vi "Main menu_3.vi"() -> ()   [LabVIEW 2022 SP3]
uses:
  <vilib>/event_ctls.llb/lveventtype.ctl
  <vilib>/Utility/file.llb/Write Delimited Spreadsheet (DBL).vi
panel:
  out "Waveform Chart 2":waveform(sgl)(graph)
  out "Waveform Chart":sgl[](graph)
  in  "# signal selec":string(combo)
  out "Close":bool
  in  "Close app":bool
  in  "?":T1(tab)
  in  "New plot":bool
  in  "Multicolumn Listbox":i32(listbox)
  in  "Close All plots":bool
  in  "CSV":bool
  in  "Start record":bool
  in  "Refresh \ntime (ms)":i32
  in  "Mode":enum32{"Item 0", "Item 1"}(radio)
  in  "Size bytes X #Traces":i32
  in  "Trace names":string(combo)
  in  "CTRL enable":bool
  in  "Save CTRL parameters":bool
  out "Total\ncontrols":i32
  in  "# Control":string(combo)
  in  "CS enable":bool
  out "Current CS status":i32
  in  "CS_IF_Params":T2 {"CS_Duty" min=0 max=1}
  out "Connected":bool
  out "Server Ping":string
  out "Saved":bool
  in  "Save conf":bool
  in  "Ping IP":bool
  in  "Port":i32
  in  "hostname":string
  in  "timeout ms":i32
  in  "Send message":bool
  in  "Process 2":i32
  in  "msj":string
  # "hostname: 127.0.0.1\nport: 8085"
  # "hostname\n131.246.75.169"
  # "Temporal for testing"
  # "Next activities:\n\n- Put preempt config in the from HW_\n- Continuos with refresh (share variable) _ temp"
  # "ctrl_if:0\nctrl: 2\nset parm: 2"
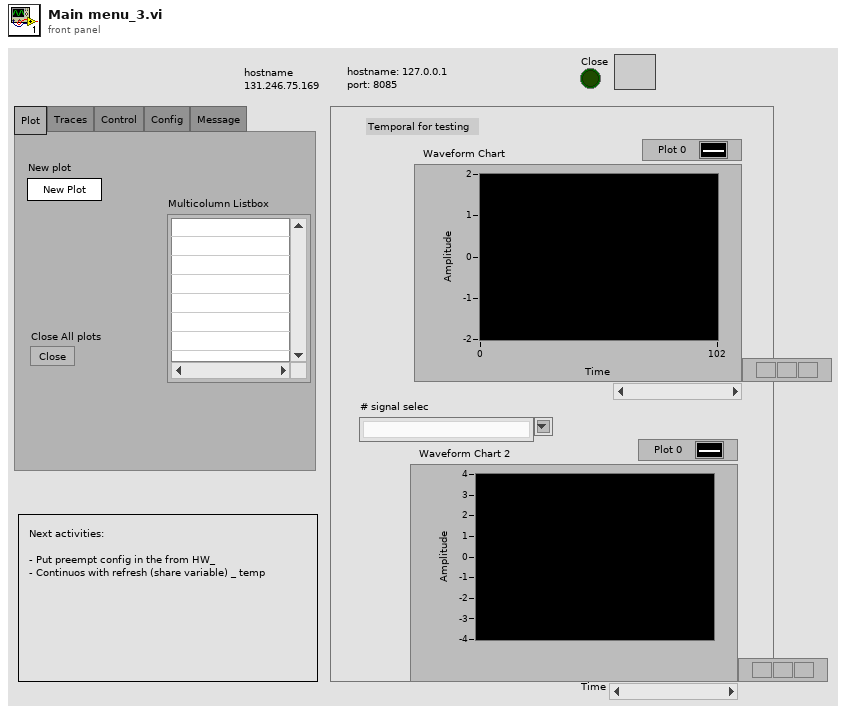
[diagram p1: front panel]
types:
  T1 = enum32{"Plot", "Traces", "Control", "Config", "Message"}
  T2 = cluster{"SET_PARAMETERS":i32, "CTLR":i32, "CS_Duty":sgl, "CTRL_IF_SET":i32}
  T3 = cluster{"Port":i32, "hostname":string, "status":bool, "timeout ms":i32, "TRACES_NAMES":string[], "Refresh time ms":i32, "Mode":enum32{"Item 0", "Item 1"}, "Start":bool, "DATA":sgl[][], "SIGNALS_NAMES":string[], "NB_SIGNALS":i32, "NB_TRACES":i32, "ID_TRACE":i32, "Mark":bool, "Counter":i32, "CTRLs_NAMES":string[], "NB_Ctrls":i32, "CS enable?":bool, "CS ID":i32}
  T4 = enum8{"Enabled", "Disabled", "Disabled and Grayed Out"}
  T5 = cluster{"TRACE_SIZE":i32, "CS_ID":i32, "TRACE ID":i32, "CMD":i32, "DATA PARAM":string}
  T6 = cluster{"TRACE_SIZE":i32, "CS_ID":i32, "TRACE ID":i32, "CMD":i32, "DATA(M)":i32}
  T7 = cluster{"timeout ms":i32, "remote port":u16, "Address":string}
  T8 = typedef "lveventtype.ctl" = enum32{"Null", "Timeout", "Annotation Menu Selection", "Annotation Menu Selection?", "App Instance Close", "App Instance Close?", "Autoscale Range Change", "Bookmark Info Change", "Cell Edit", "Cell Edit?", "Cursor Grab", "Cursor Grab?", "Cursor Menu Selection", "Cursor Menu Selection?", "Cursor Move", "Cursor Release", "Data Change", "Direction Change", "Display State Change", "Drag Ended", "Drag Enter", "Drag Leave", "Drag Over", "Drag Source Update", "Drag Starting", "Drag Starting?", "Drop", "Exec State Change", "Key Down", "Key Down?", "Key Repeat", "Key Repeat?", "Key Up", "Listbox Double Click", "Menu Activation?", "Menu Selection (App)", "Menu Selection? (App)", "Menu Selection (User)", "Mouse Down", "Mouse Down?", "Mouse Enter", "Mouse Leave", "Mouse Move", "Mouse Up", "Mouse Wheel", "NI Security User Change (App)", "Pane Size", "Panel Close", "Panel Close?", "Panel Resize", "Plot Attribute Change", "Scale Range Change", "Shortcut Menu Activation?", "Shortcut Menu Selection (App)", "Shortcut Menu Selection? (App)", "Shortcut Menu Selection (User)", "Tree Double Click", "Tree Drag", "Tree Drag?", "Tree Drop", "Tree Drop?", "Tree Item Close", "Tree Item Close?", "Tree Item Open", "Tree Item Open?", "User Event", "Value Change"}
  T9 = enum16{"open", "replace", "create", "open or create", "replace or create", "replace or create with confirmation"}
  T10 = enum16{"big-endian, network order", "native, host order", "little-endian"}
  T11 = cluster{"SIZE":i32, " TRACE DATA":sgl[], "TRACE_SIZE":i32, "NB_TRACES":i32, "NB_TRACED_SIGNALS":i32, "NAMES TRACED SIGNALS":string[], "NAMES TRACES":string[], "CS STATUS":i32, "NB_CSs":i32, "NAMES CSs":string[], "DATA (M)":sgl[], "CMD":i32}
  T12 = enum32{"invalid app kind", "Development System", "Run Time System", "Student Edition", "Embedded LabVIEW", "Evaluation", "Custom"}
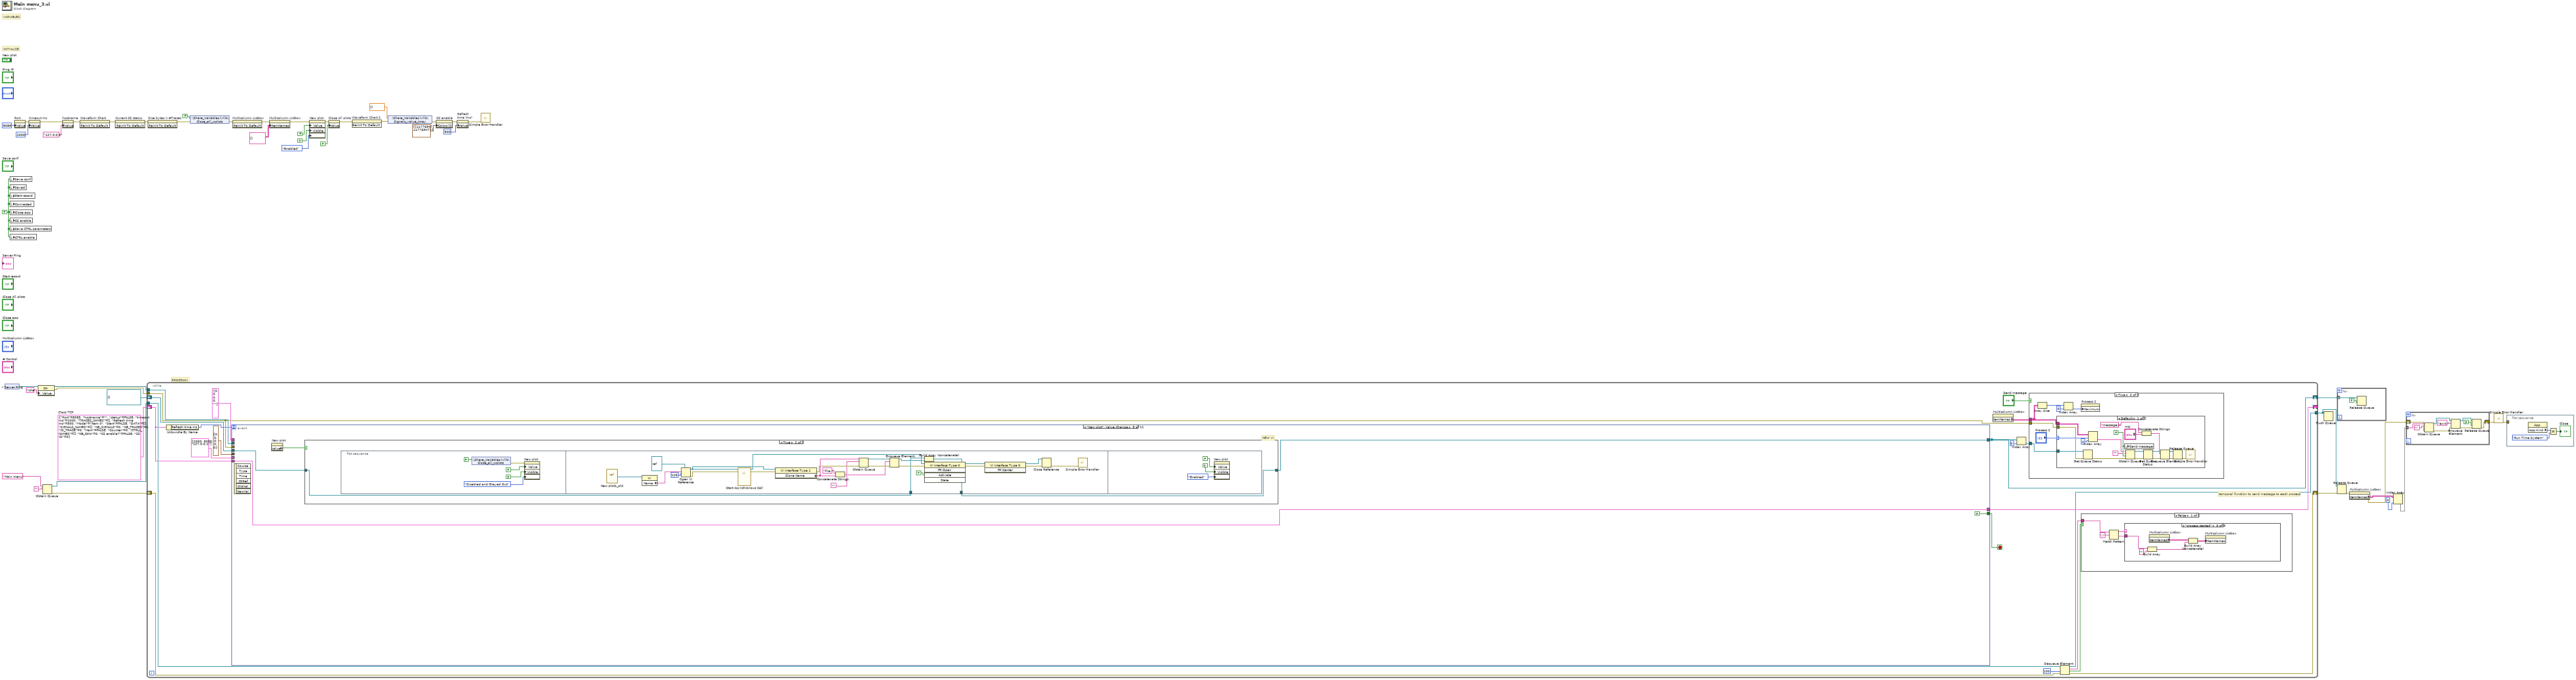
[diagram p0: block diagram]
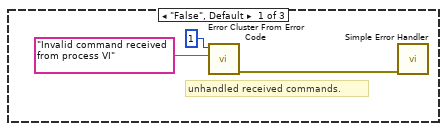
[diagram p4: hidden frame]
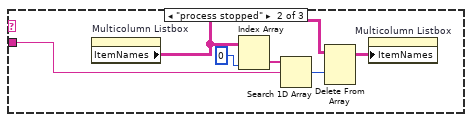
[diagram p5: hidden frame]
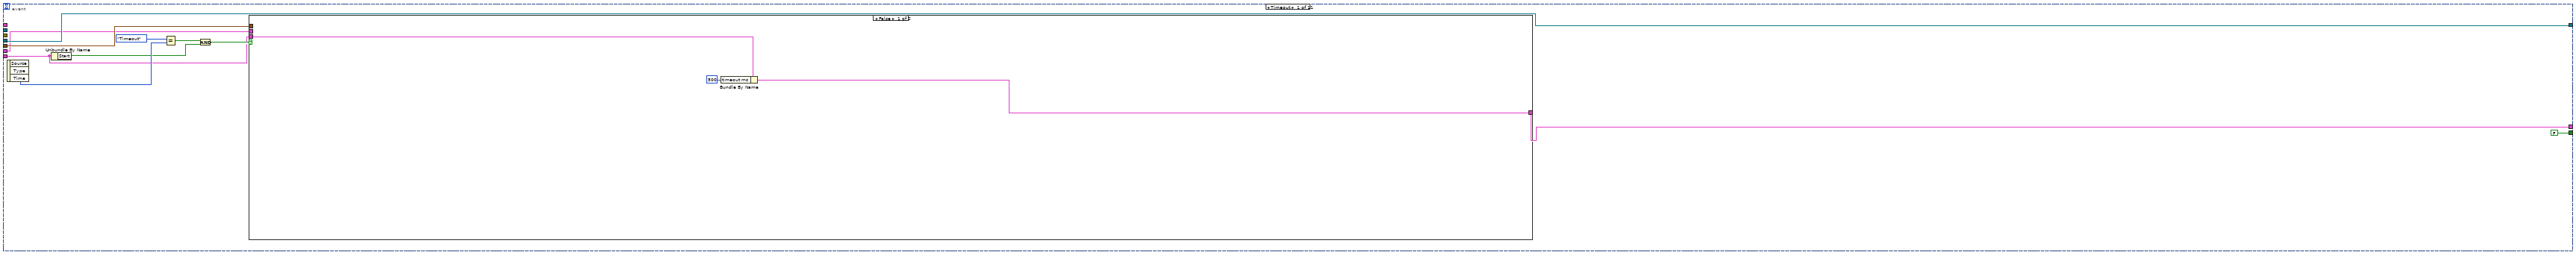
[diagram p7: hidden frame]
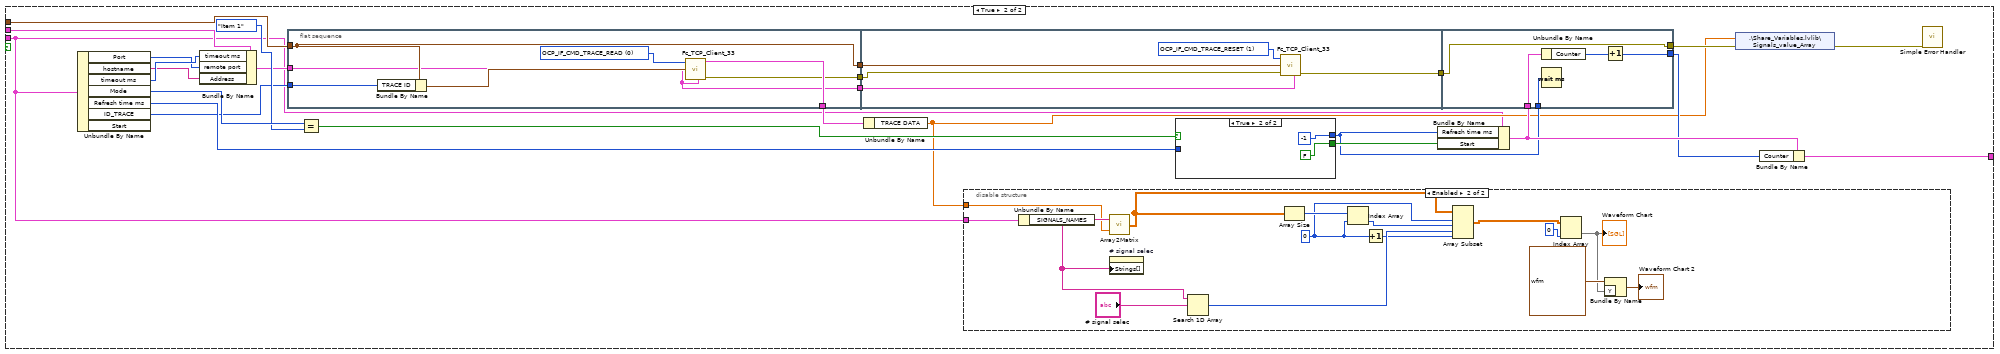
[diagram p8: hidden frame]
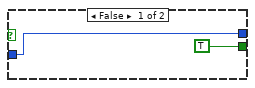
[diagram p10: hidden frame]
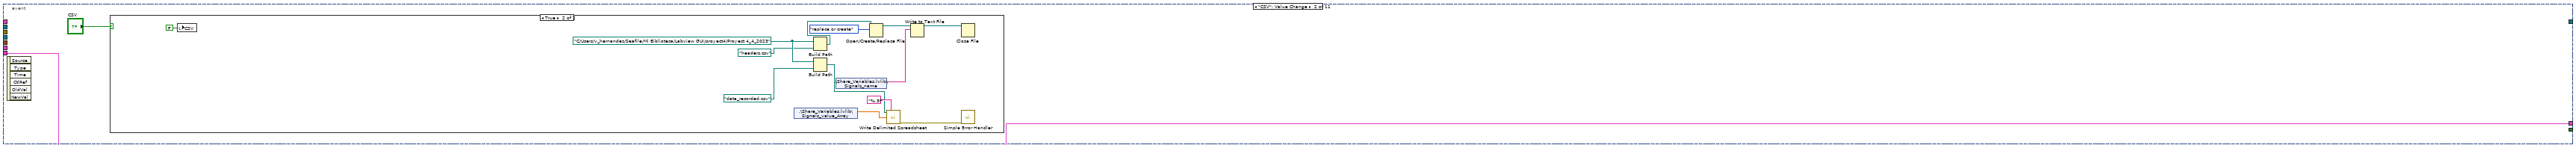
[diagram p11: hidden frame]
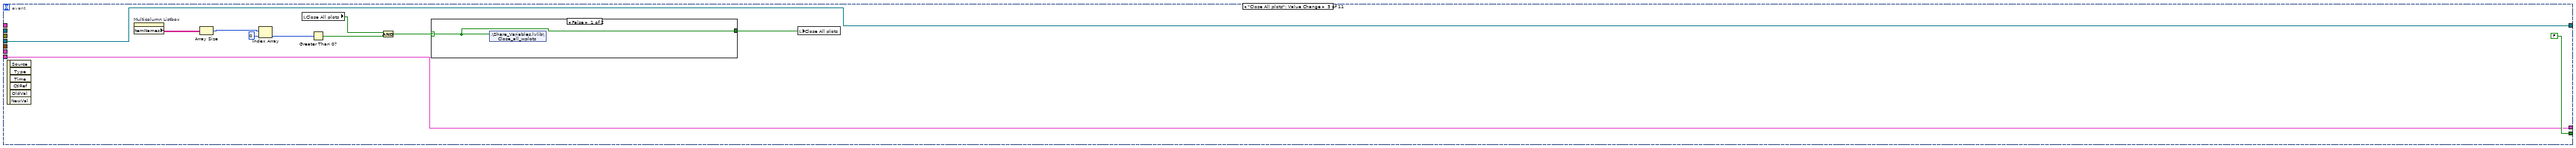
[diagram p13: hidden frame]
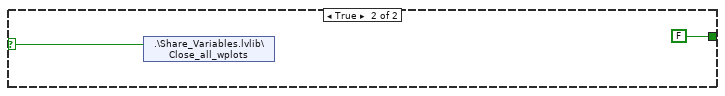
[diagram p14: hidden frame]
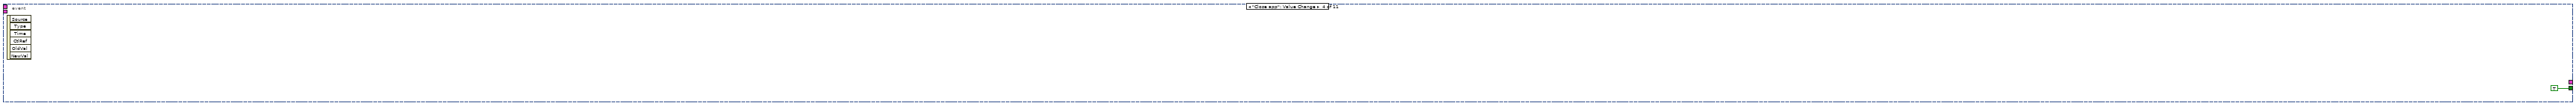
[diagram p15: hidden frame]
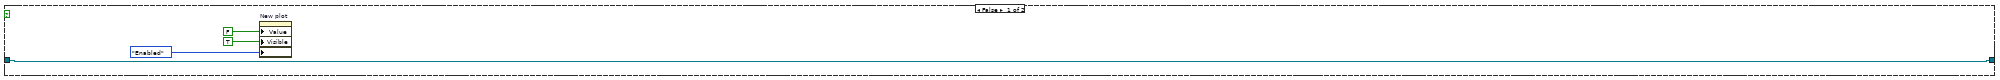
[diagram p16: hidden frame]
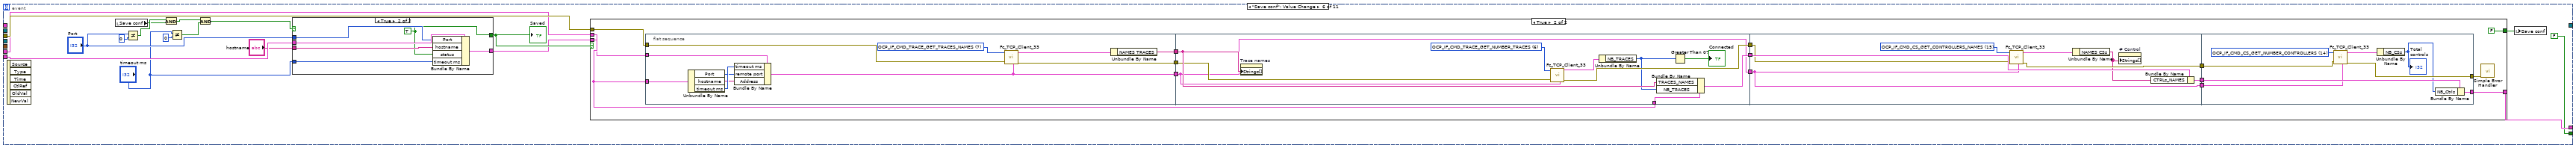
[diagram p17: hidden frame]
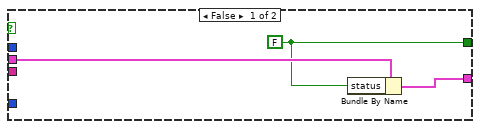
[diagram p19: hidden frame]
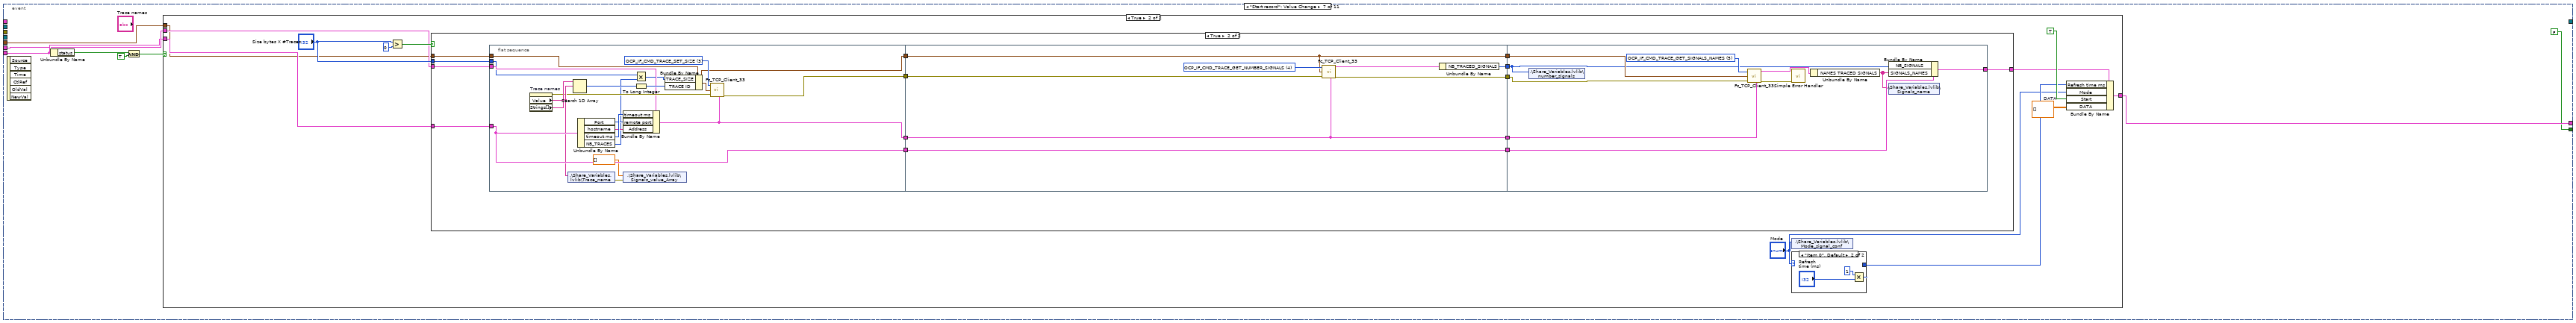
[diagram p20: hidden frame]
diagram:
  w26 = T3 {"Port"=8085, "hostname"="", "status"=FALSE, "timeout ms"=1000, "TRACES_NAMES"=[], "Refresh time ms"=500, "Mode"=enum."Item 0", "Start"=FALSE, "DATA"=[], "SIGNALS_NAMES"=[], "NB_SIGNALS"=0, "NB_TRACES"=0, "ID_TRACE"=0, "Mark"=FALSE, "Counter"=0, "CTRLs_NAMES"=[], "NB_Ctrls"=0, "CS enable?"=FALSE, "CS ID"=0}  # Class TCP
  w10 = FALSE ("Save conf")
  # "PROGRAM"
  # "INITIALIZE"
  # "VARIABLES"
  n1 = control-ref of="Server Ping"() -> (w23:refnum<vi>)
  n2 = local write "Save conf"(w10) -> ()
  n3 = local write "Saved"(w10) -> ()
  n4 = local write "Start record"(w10) -> ()
  n5 = local write "Connected"(w10) -> ()
  n6 = local write "Close app"(w10) -> ()
  n7 = local write "CS enable"(w10) -> ()
  n8 = local write "Save CTRL parameters"(w10) -> ()
  n9 = local write "CTRL enable"(w10) -> ()
  n10 = property on="Port" class="DigNum (strict)"("Value"=8085) -> (error out=w21:errorcluster)  [unwired: 2 in, 1 out]
  n11 = property on="timeout ms" class="DigNum (strict)"(error in=w21, "Value"=2000 ("timeout ms")) -> (error out=w17:errorcluster)  [unwired: 1 in, 1 out]
  n12 = property class="Str"(reference=w23, "Value"="Idle" ("Ping status")) -> (reference out=w25:refnum<vi>, error out=w24:errorcluster)  [unwired: 1 in]
  n13 = Obtain Queue(name (unnamed)="Main menu", element data type="") -> (queue out=w41:refnum<queue>, error out=w39:errorcluster)  [unwired: 3 in, 1 out]
  n14 = property on="hostname" class="Str"(error in=w17, "Value"="127.0.0.1" ("hostname")) -> (error out=w9:errorcluster)  [unwired: 1 in, 1 out]
  n15 = invoke on="Waveform Chart" class="WFChart (strict)" method="Reinit To Default"(error in=w9) -> (error out=w8:errorcluster)  [unwired: 2 in, 2 out]
  n16 = invoke on="Current CS status" class="DigNum (strict)" method="Reinit To Default"(error in=w8) -> (error out=w15:errorcluster)  [unwired: 2 in, 2 out]
  n17 = while {
    shift-right: [w53] -> w45
    shift-left: refnum<queue>[] [] -> [w69]
    tunnel: w41 -> [w68]
    tunnel: [w65] -> w31
    shift-right: [w58] -> w40
    shift-left: w39 -> [w64]
    shift-right: [w62] -> _
    shift-left: w26 -> [w60]
    tunnel: w25 -> [w61]
    tunnel: w24 -> [w55]
    stop <- w70 stop-if-true
    # "temporal function to send message to each process"
    n18 = Unbundle By Name(w60) -> ("Refresh time ms"=w59:i32)
    n19 = event shown="[4] \"New plot\": Value Change" {
      selector: _ -> [_ _ _ _ _ _ _ _ _ _ _]
      dyn-events: _ -> [_ _ _ _ _ _ _ _ _ _ _]
      timeout: w59 -> [_ _ _ _ _ _ _ _ _ _ _]
      tunnel: [FALSE ("f") _ FALSE ("f") TRUE ("f") FALSE ("f") FALSE ("f") FALSE ("f") FALSE ("f") _ _ _] -> w70
      tunnel: [w125 _ w215 _ w223 _ _ _ _ _ _] -> w53
      tunnel: w69 -> [w125 _ w215 _ w222 _ _ _ _ _ _]
      tunnel: [w118 w190 w205 _ w220 w271 w349 w423 w466 w531 w582] -> w62
      tunnel: w60 -> [w119 w190 w205 _ w220 w279 w350 w423 w465 w531 w582]
      tunnel: w61 -> [_ _ _ _ _ _ _ _ _ _ _]
      tunnel: w55 -> [_ _ _ _ _ w274 _ _ _ w532 w583]
      tunnel: T7 {"timeout ms"=2000, "remote port"=8085, "Address"="127.0.0.1"} ("Comunication Cluster") -> [w115 _ _ _ _ w264 w346 w427 w475 w528 w581]
      tunnel: T6 {"TRACE_SIZE"=0, "CS_ID"=0, "TRACE ID"=0, "CMD"=0, "DATA(M)"=0} ("Input Cluster") -> [w116 _ _ _ _ _ w345 w424 w474 _ _]
      tunnel: T5 {"TRACE_SIZE"=0, "CS_ID"=0, "TRACE ID"=0, "CMD"=0, "DATA PARAM"=""} ("Input Cluster") -> [_ _ _ _ _ _ _ _ _ w523 w576]
      event Timeout {
        n20 = event-data() -> ("Type"=w123:T8)  [unwired: 1 in, 2 out]
        n21 = Unbundle By Name(w119) -> ("Start"=w121:bool)
        n22 = Equal?(x=lveventtype."Timeout" ("Type"), y=w123) -> (x = y?=w122:bool)
        n23 = And(x=w122, y=w121) -> (x .and. y?=w120:bool)
        n24 = case shown="False" w120 {
          tunnel: w119 -> [w128 w129]
          tunnel: [w127 w143] -> w118
          tunnel: w116 -> [_ w132]
          tunnel: w115 -> [_ w131]
          frame False {
            n25 = Bundle By Name(cluster=w128, "timeout ms"=500) -> (w127:T3)
          }
          frame True {
            n26 = Unbundle By Name(w129) -> ("Port"=w137:i32, "hostname"=w136:string, "timeout ms"=w138:i32, "Mode"=w153:enum32{"Item 0", "Item 1"}, "Refresh time ms"=w150:i32, "ID_TRACE"=w147:i32)  [unwired: 1 out]
            n27 = Bundle By Name(cluster=w131, "timeout ms"=w138, "remote port"=w137, "Address"=w136) -> (w135:T7)
            n28 = flat-sequence {
              tunnel: w147 -> [w171]
              tunnel: [w175] -> w146
              tunnel: [w174] -> w145
              tunnel: w132 -> [w170]
              tunnel: [w170] -> w140
              tunnel: [w169] -> w139
              tunnel: w135 -> [w169]
              tunnel: w145 -> [w180]
              tunnel: w140 -> [w179]
              tunnel: w139 -> [w178]
              tunnel: [w176] -> w134
              tunnel: w144 -> [w185]
              tunnel: [w183] -> w142
              tunnel: w141 -> [w182]
              tunnel: w134 -> [w181]
              tunnel: [w181] -> w133
              frame #0 {
                w173 = 0 items=["OCP_IF_CMD_TRACE_READ", "OCP_IF_CMD_TRACE_RESET", "OCP_IF_CMD_TRACE_GET_SIZE", "OCP_IF_CMD_TRACE_SET_SIZE", "OCP_IF_CMD_TRACE_GET_NUMBER_SIGNALS", "OCP_IF_CMD_TRACE_GET_SIGNALS_NAMES", "OCP_IF_CMD_TRACE_GET_NUMBER_TRACES", "OCP_IF_CMD_TRACE_GET_TRACES_NAMES", "OCP_IF_CMD_TRACE_GET_ADDRESS", "OCP_IF_CMD_CS_STATUS", "OCP_IF_CMD_CS_ENABLE", "OCP_IF_CMD_CS_DISABLE", "OCP_IF_CMD_CS_CONTROLLER_IF", "OCP_IF_CMD_CS_HARDWARE_IF", "OCP_IF_CMD_CS_GET_NUMBER_CONTROLLERS", "OCP_IF_CMD_CS_GET_CONTROLLERS_NAMES", "OCP_IF_CMD_PLATFORM_ID", "OCP_IF_CMD_PLATFORM_IF", "OCP_IF_CMD_OPIL_UPDATE_MEASUREMENTS", "OCP_IF_CMD_OPIL_UPDATE_SIM_DATA", "OCP_IF_CMD_OPIL_RUN_CONTROL", "OCP_IF_CMD_OPIL_INITIALIZE_CONTROL", "OCP_IF_CMD_OPIL_GET_CONTROL", "OCP_IF_CMD_OPIL_GET_CONTROLLER_DATA", "OCP_IF_CMD_END"] ("CMD")
                n29 = Bundle By Name(cluster=w170, "TRACE ID"=w171) -> (w172:T6)
                n30 = call "Fc_TCP_Client_33.vi"("CMD"=w173, "Input Cluster"=w172, "Comunication Cluster"=w169) -> ("Output cluster"=w175:T11, "error out"=w174:errorcluster)  [unwired: 5 in, 1 out]
              }
              frame #1 {
                w177 = 1 items=["OCP_IF_CMD_TRACE_READ", "OCP_IF_CMD_TRACE_RESET", "OCP_IF_CMD_TRACE_GET_SIZE", "OCP_IF_CMD_TRACE_SET_SIZE", "OCP_IF_CMD_TRACE_GET_NUMBER_SIGNALS", "OCP_IF_CMD_TRACE_GET_SIGNALS_NAMES", "OCP_IF_CMD_TRACE_GET_NUMBER_TRACES", "OCP_IF_CMD_TRACE_GET_TRACES_NAMES", "OCP_IF_CMD_TRACE_GET_ADDRESS", "OCP_IF_CMD_CS_STATUS", "OCP_IF_CMD_CS_ENABLE", "OCP_IF_CMD_CS_DISABLE", "OCP_IF_CMD_CS_CONTROLLER_IF", "OCP_IF_CMD_CS_HARDWARE_IF", "OCP_IF_CMD_CS_GET_NUMBER_CONTROLLERS", "OCP_IF_CMD_CS_GET_CONTROLLERS_NAMES", "OCP_IF_CMD_PLATFORM_ID", "OCP_IF_CMD_PLATFORM_IF", "OCP_IF_CMD_OPIL_UPDATE_MEASUREMENTS", "OCP_IF_CMD_OPIL_UPDATE_SIM_DATA", "OCP_IF_CMD_OPIL_RUN_CONTROL", "OCP_IF_CMD_OPIL_INITIALIZE_CONTROL", "OCP_IF_CMD_OPIL_GET_CONTROL", "OCP_IF_CMD_OPIL_GET_CONTROLLER_DATA", "OCP_IF_CMD_END"] ("CMD")
                n31 = call "Fc_TCP_Client_33.vi"("CMD"=w177, "Input Cluster"=w179, "error in (no error)"=w180, "Comunication Cluster"=w178) -> ("error out"=w176:errorcluster)  [unwired: 4 in, 2 out]
              }
              frame #2 {
                n32 = Unbundle By Name(w185) -> ("Counter"=w184:i32)
                n33 = Wait (ms)(milliseconds to wait=w182) -> ()  [unwired: 1 out]
                n34 = Increment(x=w184) -> (x+1=w183:i32)
              }
            }
            n35 = Equal?(x=w153, y=enum32{"Item 0", "Item 1"}."Item 1" ("Mode")) -> (x = y?=w151:bool)
            n36 = Unbundle By Name(w146) -> ("TRACE DATA"=w130:sgl[])
            n37 = disable-structure shown="Enabled" {
              disable-tunnel: w130 -> [_ w164]
              disable-tunnel: w129 -> [_ w168]
              frame Disabled {
              }
              frame Enabled {
                w159 = 0 ("index")
                n38 = Unbundle By Name(w168) -> ("SIGNALS_NAMES"=w166:string[])
                n39 = call "Array2Matrix.vi"("Array"=w164, "Header"=w166) -> ("Array2D"=w163:sgl[][])
                n40 = property on="# signal selec" class="CmbBox"("Strings[]"=w166) -> ()  [unwired: 2 in, 2 out]
                n41 = Search 1D Array(1D array=w166, element="# signal selec") -> (index of element=w165:i32)  [unwired: 1 in]
                n42 = Array Size(array=w163) -> (size(s)=w162:i32[])
                n43 = Index Array(array=w162, index=w159) -> (element=w161:i32)
                n44 = Increment(x=w159) -> (x+1=w158:i32)
                n45 = Array Subset(array=w163, index (row)=w159, length (row)=w161, index (col)=w165, length (col)=w158) -> (w157:sgl[][])
                n46 = Index Array(array=w157, index (col)=0 ("disabled index (col)")) -> (element=w155:sgl[])  [unwired: 1 in]
                "Waveform Chart" <- w155
                n47 = Bundle By Name(cluster=waveform(sgl) {"t0"=timestamp(0 s since 1904-01-01), "dt"=1.0, "Y"=[]} ("waveform"), "Y"=w155) -> (→"Waveform Chart 2":waveform(sgl))
              }
            }
            n48 = case shown="True" w151 {
              tunnel: [TRUE FALSE] -> w149
              tunnel: [w186 i8 -1 ("t")] -> w141
              tunnel: w150 -> [w186 _]
              frame False {
              }
              frame True {
              }
            }
            n49 = Bundle By Name(cluster=w129, "Refresh time ms"=w141, "Start"=w149) -> (w144:T3)
            n50 = shared-variable ".\\Share_Variables.lvlib\\Signals_value_Array"(w130, error in=w133) -> (error out=w148:errorcluster)
            n51 = Bundle By Name(cluster=w144, "Counter"=w142) -> (w143:T3)
            n52 = call <vilib>:"Simple Error Handler.vi"("error in (no error)"=w148) -> ()  [unwired: 4 in, 5 out]
          }
        }
      }
      event "CSV": Value Change {
        n53 = event-data() -> ()  [unwired: 1 in, 6 out]
        n54 = case shown="True" "CSV" {
          frame False {
          }
          frame True {
            w199 = path "C:/Users/v_hernandez/Seafile/Mi Biblioteca/Labview GUI/proyect4/Proyect 4_4_2023" ("base path")
            n55 = local write "CSV"(FALSE ("CSV")) -> ()
            n56 = shared-variable ".\\Share_Variables.lvlib\\Signals_value_Array"() -> (w201:dbl[])  [unwired: 1 in, 1 out]
            n57 = Build Path(base path=w199, name or relative path=path "headers.csv") -> (appended path=w197:path)
            n58 = Build Path(base path=w199, name or relative path=path "data_recorded.csv") -> (appended path=w200:path)
            n59 = shared-variable ".\\Share_Variables.lvlib\\Signals_name"() -> (w194:string[])  [unwired: 1 in, 1 out]
            n60 = Open/Create/Replace File(file path (use dialog)=w197, operation (0:open)=T9."replace or create") -> (refnum out=w195:refnum<file>)  [unwired: 4 in, 2 out]
            n61 = call-poly <vilib>:"Write Delimited Spreadsheet.vi"("file path (dialog if empty)"=w200, "format (%.3f)"="%.3f", "1D data"=w201) -> ("error out"=w202:errorcluster)  [unwired: 11 in, 1 out]
            n62 = Write to Text File(file (use dialog)=w195, text=w194) -> (refnum out=w193:refnum<file>)  [unwired: 2 in, 2 out]
            n63 = Close File(refnum=w193) -> ()  [unwired: 1 in, 2 out]
            n64 = call <vilib>:"Simple Error Handler.vi"("error in (no error)"=w202) -> ()  [unwired: 4 in, 5 out]
          }
        }
      }
      event "Close All plots": Value Change {
        n65 = event-data() -> ()  [unwired: 1 in, 6 out]
        n66 = property on="Multicolumn Listbox" class="MCListbox (strict)"() -> ("ItemNames"=w209:string[][])  [unwired: 2 in, 2 out]
        n67 = Array Size(array=w209) -> (size(s)=w213:i32[])
        n68 = Index Array(array=w213, index=0) -> (element=w211:i32)
        n69 = local read "Close All plots"() -> (w208:bool)
        n70 = Greater Than 0?(x=w211) -> (x > 0?=w206:bool)
        n71 = And(x=w208, y=w206) -> (x .and. y?=w207:bool)
        n72 = case shown="False" w207 {
          selector: w207 -> [w216 w217]
          tunnel: [w216 FALSE] -> w210
          frame False {
            n73 = shared-variable ".\\Share_Variables.lvlib\\Close_all_wplots"(w216) -> ()  [unwired: 1 in, 1 out]
          }
          frame True {
            n74 = shared-variable ".\\Share_Variables.lvlib\\Close_all_wplots"(w217) -> ()  [unwired: 1 in, 1 out]
          }
        }
        n75 = local write "Close All plots"(w210) -> ()
      }
      event "Close app": Value Change {
        n76 = event-data() -> ()  [unwired: 1 in, 6 out]
      }
      event "New plot": Value Change {
        # "NEW VI"
        n77 = event-data() -> ()  [unwired: 1 in, 6 out]
        n78 = property on="New plot" class="Bool (strict)"() -> ("Value"=w224:bool)  [unwired: 2 in, 2 out]
        n79 = case shown="True" w224 {
          tunnel: [w225 w230] -> w223
          tunnel: w222 -> [w225 w229]
          frame False {
            n80 = property on="New plot" class="Bool (strict)"("Value"=FALSE ("New plot"), "Visible"=TRUE, "DisabledEnum"=T4."Enabled" ("Disabled")) -> ()  [unwired: 2 in, 2 out]
          }
          frame True {
            n81 = flat-sequence {
              tunnel: [w241] -> w230
              tunnel: w229 -> [w240]
              frame #0 {
                n82 = shared-variable ".\\Share_Variables.lvlib\\Close_all_wplots"(FALSE ("Close_all_wplots")) -> (error out=w231:errorcluster)  [unwired: 1 in]
                n83 = property on="New plot" class="Bool (strict)"(error in=w231, "Value"=FALSE ("New plot"), "Visible"=FALSE, "DisabledEnum"=T4."Disabled and Grayed Out" ("Disabled")) -> ()  [unwired: 1 in, 2 out]
              }
              frame #1 {
                n84 = vi-ref "New plot1_old.vi"() -> (w254:refnum<vi>)
                n85 = property class="VI"(reference=w254) -> ("Name"=w260:string)  [unwired: 1 in, 2 out]
                n86 = Open VI Reference(type specifier VI Refnum (for type only)=refnum<vi> refnum, vi path=w260, options=128) -> (vi reference=w251:refnum<vi>, error out=w256:errorcluster)  [unwired: 3 in]
                n87 = call-by-ref "Start Asynchronous Call"(reference=w251, error in=w256) -> (reference out=w255:refnum<vi>, error out=w245:errorcluster)  [unwired: 1 in, 1 out]
                n88 = property class="VI Interface Type 1"(reference=w251, error in=w245) -> (error out=w246:errorcluster, "Clone Name"=w248:string)  [unwired: 1 out]
                n89 = Concatenate Strings("file::" ("string"), w248) -> (w239:string)
                n90 = Obtain Queue(name (unnamed)=w248, element data type="", error in (no error)=w246) -> (queue out=w247:refnum<queue>, error out=w244:errorcluster)  [unwired: 2 in, 1 out]
                n91 = Enqueue Element(queue=w247, element=w239, error in (no error)=w244) -> (queue out=w242:refnum<queue>, error out=w243:errorcluster)  [unwired: 1 in, 1 out]
                n92 = Build Array (concatenate)(w240, w242) -> (w241:refnum<queue>[])
                n93 = invoke class="VI Interface Type 0" method="FP.Open"(reference=w255, error in=w243, "Activate"=TRUE ("Activate?")) -> (reference out=w253:refnum<vi>, error out=w238:errorcluster)  [unwired: 2 in, 3 out]
                n94 = invoke class="VI Interface Type 0" method="FP.Center"(reference=w253, error in=w238) -> (reference out=w252:refnum<vi>, error out=w237:errorcluster)  [unwired: 1 in, 1 out]
                n95 = Close Reference(reference=w252, error in (no error)=w237) -> (error out=w236:errorcluster)
                n96 = call <vilib>:"Simple Error Handler.vi"("error in (no error)"=w236) -> ()  [unwired: 4 in, 5 out]
              }
              frame #2 {
                n97 = property on="New plot" class="Bool (strict)"("Value"=FALSE ("Value (Signaling)"), "Visible"=TRUE, "DisabledEnum"=T4."Enabled" ("Disabled")) -> ()  [unwired: 2 in, 2 out]
              }
            }
          }
        }
      }
      event "Save conf": Value Change {
        n98 = event-data() -> ()  [unwired: 1 in, 6 out]
        n99 = local read "Save conf"() -> (w276:bool)
        n100 = Not Equal?(x="Port", y=0) -> (x != y?=w280:bool)
        n101 = And(x=w280, y=w276) -> (x .and. y?=w266:bool)
        n102 = Not Equal?(x="timeout ms", y=0) -> (x != y?=w268:bool)
        n103 = And(x=w266, y=w268) -> (x .and. y?=w267:bool)
        n104 = case shown="True" w267 {
          tunnel: [w336 w341] -> w275
          tunnel: "Port" -> [_ w343]
          tunnel: "hostname" -> [_ w342]
          tunnel: [w338 w339] -> w272
          tunnel: w279 -> [w337 w344]
          tunnel: "timeout ms" -> [_ w340]
          frame False {
            w336 = FALSE
            n105 = Bundle By Name(cluster=w337, "status"=w336) -> (w338:T3)
          }
          frame True {
            w341 = TRUE
            n106 = Bundle By Name(cluster=w344, "Port"=w343, "hostname"=w342, "status"=w341, "timeout ms"=w340) -> (w339:T3)
          }
        }
        "Saved" <- w275
        n107 = case shown="True" w275 {
          selector: w275 -> [w282 _]
          tunnel: w274 -> [_ w286]
          tunnel: [w282 FALSE] -> w273
          tunnel: w272 -> [w283 w297]
          tunnel: [w283 w296] -> w271
          tunnel: w264 -> [_ w284]
          frame False {
          }
          frame True {
            n108 = flat-sequence {
              tunnel: w297 -> [w309]
              tunnel: [w303] -> w295
              tunnel: [w302] -> w294
              tunnel: [w301] -> w293
              tunnel: w286 -> [w300]
              tunnel: w284 -> [w299]
              tunnel: w297 -> [w319]
              tunnel: w295 -> [w317]
              tunnel: w294 -> [w316]
              tunnel: w293 -> [w312]
              tunnel: [w318] -> w292
              tunnel: [w313] -> w290
              tunnel: [w312] -> w289
              tunnel: w292 -> [w327]
              tunnel: [w321] -> w291
              tunnel: w290 -> [w326]
              tunnel: w289 -> [w323]
              tunnel: [w324] -> w288
              tunnel: [w323] -> w287
              tunnel: [w331] -> w296
              tunnel: w291 -> [w335]
              tunnel: w288 -> [w334]
              tunnel: w287 -> [w333]
              tunnel: [w329] -> w285
              frame #0 {
                w308 = 7 items=["OCP_IF_CMD_TRACE_READ", "OCP_IF_CMD_TRACE_RESET", "OCP_IF_CMD_TRACE_GET_SIZE", "OCP_IF_CMD_TRACE_SET_SIZE", "OCP_IF_CMD_TRACE_GET_NUMBER_SIGNALS", "OCP_IF_CMD_TRACE_GET_SIGNALS_NAMES", "OCP_IF_CMD_TRACE_GET_NUMBER_TRACES", "OCP_IF_CMD_TRACE_GET_TRACES_NAMES", "OCP_IF_CMD_TRACE_GET_ADDRESS", "OCP_IF_CMD_CS_STATUS", "OCP_IF_CMD_CS_ENABLE", "OCP_IF_CMD_CS_DISABLE", "OCP_IF_CMD_CS_CONTROLLER_IF", "OCP_IF_CMD_CS_HARDWARE_IF", "OCP_IF_CMD_CS_GET_NUMBER_CONTROLLERS", "OCP_IF_CMD_CS_GET_CONTROLLERS_NAMES", "OCP_IF_CMD_PLATFORM_ID", "OCP_IF_CMD_PLATFORM_IF", "OCP_IF_CMD_OPIL_UPDATE_MEASUREMENTS", "OCP_IF_CMD_OPIL_UPDATE_SIM_DATA", "OCP_IF_CMD_OPIL_RUN_CONTROL", "OCP_IF_CMD_OPIL_INITIALIZE_CONTROL", "OCP_IF_CMD_OPIL_GET_CONTROL", "OCP_IF_CMD_OPIL_GET_CONTROLLER_DATA", "OCP_IF_CMD_END"] ("CMD")
                n109 = Unbundle By Name(w309) -> ("Port"=w305:i32, "hostname"=w304:string, "timeout ms"=w306:i32)
                n110 = Bundle By Name(cluster=w299, "timeout ms"=w306, "remote port"=w305, "Address"=w304) -> (w301:T7)
                n111 = call "Fc_TCP_Client_33.vi"("CMD"=w308, "error in (no error)"=w300, "Comunication Cluster"=w301) -> ("Output cluster"=w307:T11, "error out"=w302:errorcluster)  [unwired: 5 in, 1 out]
                n112 = Unbundle By Name(w307) -> ("NAMES TRACES"=w303:string[])
              }
              frame #1 {
                w315 = 6 items=["OCP_IF_CMD_TRACE_READ", "OCP_IF_CMD_TRACE_RESET", "OCP_IF_CMD_TRACE_GET_SIZE", "OCP_IF_CMD_TRACE_SET_SIZE", "OCP_IF_CMD_TRACE_GET_NUMBER_SIGNALS", "OCP_IF_CMD_TRACE_GET_SIGNALS_NAMES", "OCP_IF_CMD_TRACE_GET_NUMBER_TRACES", "OCP_IF_CMD_TRACE_GET_TRACES_NAMES", "OCP_IF_CMD_TRACE_GET_ADDRESS", "OCP_IF_CMD_CS_STATUS", "OCP_IF_CMD_CS_ENABLE", "OCP_IF_CMD_CS_DISABLE", "OCP_IF_CMD_CS_CONTROLLER_IF", "OCP_IF_CMD_CS_HARDWARE_IF", "OCP_IF_CMD_CS_GET_NUMBER_CONTROLLERS", "OCP_IF_CMD_CS_GET_CONTROLLERS_NAMES", "OCP_IF_CMD_PLATFORM_ID", "OCP_IF_CMD_PLATFORM_IF", "OCP_IF_CMD_OPIL_UPDATE_MEASUREMENTS", "OCP_IF_CMD_OPIL_UPDATE_SIM_DATA", "OCP_IF_CMD_OPIL_RUN_CONTROL", "OCP_IF_CMD_OPIL_INITIALIZE_CONTROL", "OCP_IF_CMD_OPIL_GET_CONTROL", "OCP_IF_CMD_OPIL_GET_CONTROLLER_DATA", "OCP_IF_CMD_END"] ("CMD")
                n113 = property on="Trace names" class="CmbBox"("Strings[]"=w317) -> ()  [unwired: 2 in, 2 out]
                n114 = call "Fc_TCP_Client_33.vi"("CMD"=w315, "error in (no error)"=w316, "Comunication Cluster"=w312) -> ("Output cluster"=w314:T11, "error out"=w313:errorcluster)  [unwired: 5 in, 1 out]
                n115 = Unbundle By Name(w314) -> ("NB_TRACES"=w311:i32)
                n116 = Bundle By Name(cluster=w319, "TRACES_NAMES"=w317, "NB_TRACES"=w311) -> (w318:T3)
                n117 = Greater Than 0?(x=w311) -> (x > 0?=→"Connected":bool)
              }
              frame #2 {
                w325 = 15 items=["OCP_IF_CMD_TRACE_READ", "OCP_IF_CMD_TRACE_RESET", "OCP_IF_CMD_TRACE_GET_SIZE", "OCP_IF_CMD_TRACE_SET_SIZE", "OCP_IF_CMD_TRACE_GET_NUMBER_SIGNALS", "OCP_IF_CMD_TRACE_GET_SIGNALS_NAMES", "OCP_IF_CMD_TRACE_GET_NUMBER_TRACES", "OCP_IF_CMD_TRACE_GET_TRACES_NAMES", "OCP_IF_CMD_TRACE_GET_ADDRESS", "OCP_IF_CMD_CS_STATUS", "OCP_IF_CMD_CS_ENABLE", "OCP_IF_CMD_CS_DISABLE", "OCP_IF_CMD_CS_CONTROLLER_IF", "OCP_IF_CMD_CS_HARDWARE_IF", "OCP_IF_CMD_CS_GET_NUMBER_CONTROLLERS", "OCP_IF_CMD_CS_GET_CONTROLLERS_NAMES", "OCP_IF_CMD_PLATFORM_ID", "OCP_IF_CMD_PLATFORM_IF", "OCP_IF_CMD_OPIL_UPDATE_MEASUREMENTS", "OCP_IF_CMD_OPIL_UPDATE_SIM_DATA", "OCP_IF_CMD_OPIL_RUN_CONTROL", "OCP_IF_CMD_OPIL_INITIALIZE_CONTROL", "OCP_IF_CMD_OPIL_GET_CONTROL", "OCP_IF_CMD_OPIL_GET_CONTROLLER_DATA", "OCP_IF_CMD_END"] ("CMD")
                n118 = call "Fc_TCP_Client_33.vi"("CMD"=w325, "error in (no error)"=w326, "Comunication Cluster"=w323) -> ("Output cluster"=w322:T11, "error out"=w324:errorcluster)  [unwired: 5 in, 1 out]
                n119 = Unbundle By Name(w322) -> ("NAMES CSs"=w320:string[])
                n120 = property on="# Control" class="CmbBox"("Strings[]"=w320) -> ()  [unwired: 2 in, 2 out]
                n121 = Bundle By Name(cluster=w327, "CTRLs_NAMES"=w320) -> (w321:T3)
              }
              frame #3 {
                w332 = 14 items=["OCP_IF_CMD_TRACE_READ", "OCP_IF_CMD_TRACE_RESET", "OCP_IF_CMD_TRACE_GET_SIZE", "OCP_IF_CMD_TRACE_SET_SIZE", "OCP_IF_CMD_TRACE_GET_NUMBER_SIGNALS", "OCP_IF_CMD_TRACE_GET_SIGNALS_NAMES", "OCP_IF_CMD_TRACE_GET_NUMBER_TRACES", "OCP_IF_CMD_TRACE_GET_TRACES_NAMES", "OCP_IF_CMD_TRACE_GET_ADDRESS", "OCP_IF_CMD_CS_STATUS", "OCP_IF_CMD_CS_ENABLE", "OCP_IF_CMD_CS_DISABLE", "OCP_IF_CMD_CS_CONTROLLER_IF", "OCP_IF_CMD_CS_HARDWARE_IF", "OCP_IF_CMD_CS_GET_NUMBER_CONTROLLERS", "OCP_IF_CMD_CS_GET_CONTROLLERS_NAMES", "OCP_IF_CMD_PLATFORM_ID", "OCP_IF_CMD_PLATFORM_IF", "OCP_IF_CMD_OPIL_UPDATE_MEASUREMENTS", "OCP_IF_CMD_OPIL_UPDATE_SIM_DATA", "OCP_IF_CMD_OPIL_RUN_CONTROL", "OCP_IF_CMD_OPIL_INITIALIZE_CONTROL", "OCP_IF_CMD_OPIL_GET_CONTROL", "OCP_IF_CMD_OPIL_GET_CONTROLLER_DATA", "OCP_IF_CMD_END"] ("CMD")
                n122 = call "Fc_TCP_Client_33.vi"("CMD"=w332, "error in (no error)"=w334, "Comunication Cluster"=w333) -> ("Output cluster"=w330:T11, "error out"=w329:errorcluster)  [unwired: 5 in, 1 out]
                n123 = Unbundle By Name(w330) -> ("NB_CSs"=w328:i32)
                "Total\ncontrols" <- w328
                n124 = Bundle By Name(cluster=w335, "NB_Ctrls"=w328) -> (w331:T3)
              }
            }
            n125 = call <vilib>:"Simple Error Handler.vi"("error in (no error)"=w285) -> ()  [unwired: 4 in, 5 out]
          }
        }
        n126 = local write "Save conf"(w273) -> ()
      }
      event "Start record": Value Change {
        n127 = event-data() -> ()  [unwired: 1 in, 6 out]
        n128 = Unbundle By Name(w350) -> ("status"=w352:bool)
        n129 = And(x=w352, y=TRUE) -> (x .and. y?=w351:bool)
        n130 = case shown="True" w351 {
          tunnel: w350 -> [w353 w359]
          tunnel: [w353 w365] -> w349
          tunnel: w346 -> [_ w356]
          tunnel: w345 -> [_ w355]
          frame False {
          }
          frame True {
            w354 = sgl[][] []  # DATA
            n131 = Greater?(x="Size bytes X #Traces", y=0) -> (0:w361:bool)
            n132 = case shown="True" w361 {
              tunnel: "Size bytes X #Traces" -> [_ w380]
              tunnel: w359 -> [w366 w379]
              tunnel: [w366 w375] -> w358
              tunnel: w356 -> [_ w368]
              tunnel: w355 -> [_ w367]
              frame False {
              }
              frame True {
                n133 = flat-sequence {
                  tunnel: w380 -> [w384]
                  tunnel: w379 -> [w400]
                  tunnel: [w396] -> w378
                  tunnel: [w400] -> w377
                  tunnel: [w389] -> w374
                  tunnel: [w388] -> w373
                  tunnel: w368 -> [w387]
                  tunnel: w367 -> [w386]
                  tunnel: w378 -> [w407]
                  tunnel: w377 -> [w408]
                  tunnel: [w408] -> w376
                  tunnel: w374 -> [w401]
                  tunnel: w373 -> [w402]
                  tunnel: [w404] -> w372
                  tunnel: [w403] -> w371
                  tunnel: [w402] -> w370
                  tunnel: [w401] -> w369
                  tunnel: w376 -> [w418]
                  tunnel: [w417] -> w375
                  tunnel: w372 -> [w409]
                  tunnel: w371 -> [w413]
                  tunnel: w370 -> [w411]
                  tunnel: w369 -> [w410]
                  frame #0 {
                    w395 = 3 items=["OCP_IF_CMD_TRACE_READ", "OCP_IF_CMD_TRACE_RESET", "OCP_IF_CMD_TRACE_GET_SIZE", "OCP_IF_CMD_TRACE_SET_SIZE", "OCP_IF_CMD_TRACE_GET_NUMBER_SIGNALS", "OCP_IF_CMD_TRACE_GET_SIGNALS_NAMES", "OCP_IF_CMD_TRACE_GET_NUMBER_TRACES", "OCP_IF_CMD_TRACE_GET_TRACES_NAMES", "OCP_IF_CMD_TRACE_GET_ADDRESS", "OCP_IF_CMD_CS_STATUS", "OCP_IF_CMD_CS_ENABLE", "OCP_IF_CMD_CS_DISABLE", "OCP_IF_CMD_CS_CONTROLLER_IF", "OCP_IF_CMD_CS_HARDWARE_IF", "OCP_IF_CMD_CS_GET_NUMBER_CONTROLLERS", "OCP_IF_CMD_CS_GET_CONTROLLERS_NAMES", "OCP_IF_CMD_PLATFORM_ID", "OCP_IF_CMD_PLATFORM_IF", "OCP_IF_CMD_OPIL_UPDATE_MEASUREMENTS", "OCP_IF_CMD_OPIL_UPDATE_SIM_DATA", "OCP_IF_CMD_OPIL_RUN_CONTROL", "OCP_IF_CMD_OPIL_INITIALIZE_CONTROL", "OCP_IF_CMD_OPIL_GET_CONTROL", "OCP_IF_CMD_OPIL_GET_CONTROLLER_DATA", "OCP_IF_CMD_END"] ("CMD")
                    n134 = property on="Trace names" class="CmbBox"() -> (error out=w391:errorcluster, "Value"=w397:string, "Strings[]"=w399:string[])  [unwired: 2 in, 1 out]
                    n135 = shared-variable ".\\Share_Variables.lvlib\\Trace_name"(w397) -> (error out=w382:errorcluster)  [unwired: 1 in]
                    n136 = Search 1D Array(1D array=w399, element=w397) -> (index of element=w398:i32)  [unwired: 1 in]
                    n137 = Unbundle By Name(w400) -> ("Port"=w393:i32, "hostname"=w392:string, "timeout ms"=w394:i32, "NB_TRACES"=w385:i32)
                    n138 = Bundle By Name(cluster=w387, "timeout ms"=w394, "remote port"=w393, "Address"=w392) -> (w388:T7)
                    n139 = shared-variable ".\\Share_Variables.lvlib\\Signals_value_Array"(dbl[] [] ("Signals_value_Array"), error in=w382) -> ()  [unwired: 1 out]
                    n140 = Multiply(x=w384, y=w385) -> (x*y=w383:i32)
                    n141 = To Long Integer(number=w398) -> (32bit integer=w390:i32)
                    n142 = Bundle By Name(cluster=w386, "TRACE_SIZE"=w383, "TRACE ID"=w390) -> (w389:T6)
                    n143 = call "Fc_TCP_Client_33.vi"("CMD"=w395, "Input Cluster"=w389, "error in (no error)"=w391, "Comunication Cluster"=w388) -> ("error out"=w396:errorcluster)  [unwired: 4 in, 2 out]
                  }
                  frame #1 {
                    w406 = 4 items=["OCP_IF_CMD_TRACE_READ", "OCP_IF_CMD_TRACE_RESET", "OCP_IF_CMD_TRACE_GET_SIZE", "OCP_IF_CMD_TRACE_SET_SIZE", "OCP_IF_CMD_TRACE_GET_NUMBER_SIGNALS", "OCP_IF_CMD_TRACE_GET_SIGNALS_NAMES", "OCP_IF_CMD_TRACE_GET_NUMBER_TRACES", "OCP_IF_CMD_TRACE_GET_TRACES_NAMES", "OCP_IF_CMD_TRACE_GET_ADDRESS", "OCP_IF_CMD_CS_STATUS", "OCP_IF_CMD_CS_ENABLE", "OCP_IF_CMD_CS_DISABLE", "OCP_IF_CMD_CS_CONTROLLER_IF", "OCP_IF_CMD_CS_HARDWARE_IF", "OCP_IF_CMD_CS_GET_NUMBER_CONTROLLERS", "OCP_IF_CMD_CS_GET_CONTROLLERS_NAMES", "OCP_IF_CMD_PLATFORM_ID", "OCP_IF_CMD_PLATFORM_IF", "OCP_IF_CMD_OPIL_UPDATE_MEASUREMENTS", "OCP_IF_CMD_OPIL_UPDATE_SIM_DATA", "OCP_IF_CMD_OPIL_RUN_CONTROL", "OCP_IF_CMD_OPIL_INITIALIZE_CONTROL", "OCP_IF_CMD_OPIL_GET_CONTROL", "OCP_IF_CMD_OPIL_GET_CONTROLLER_DATA", "OCP_IF_CMD_END"] ("CMD")
                    n144 = call "Fc_TCP_Client_33.vi"("CMD"=w406, "Input Cluster"=w401, "error in (no error)"=w407, "Comunication Cluster"=w402) -> ("Output cluster"=w405:T11, "error out"=w403:errorcluster)  [unwired: 4 in, 1 out]
                    n145 = Unbundle By Name(w405) -> ("NB_TRACED_SIGNALS"=w404:i32)
                  }
                  frame #2 {
                    w412 = 5 items=["OCP_IF_CMD_TRACE_READ", "OCP_IF_CMD_TRACE_RESET", "OCP_IF_CMD_TRACE_GET_SIZE", "OCP_IF_CMD_TRACE_SET_SIZE", "OCP_IF_CMD_TRACE_GET_NUMBER_SIGNALS", "OCP_IF_CMD_TRACE_GET_SIGNALS_NAMES", "OCP_IF_CMD_TRACE_GET_NUMBER_TRACES", "OCP_IF_CMD_TRACE_GET_TRACES_NAMES", "OCP_IF_CMD_TRACE_GET_ADDRESS", "OCP_IF_CMD_CS_STATUS", "OCP_IF_CMD_CS_ENABLE", "OCP_IF_CMD_CS_DISABLE", "OCP_IF_CMD_CS_CONTROLLER_IF", "OCP_IF_CMD_CS_HARDWARE_IF", "OCP_IF_CMD_CS_GET_NUMBER_CONTROLLERS", "OCP_IF_CMD_CS_GET_CONTROLLERS_NAMES", "OCP_IF_CMD_PLATFORM_ID", "OCP_IF_CMD_PLATFORM_IF", "OCP_IF_CMD_OPIL_UPDATE_MEASUREMENTS", "OCP_IF_CMD_OPIL_UPDATE_SIM_DATA", "OCP_IF_CMD_OPIL_RUN_CONTROL", "OCP_IF_CMD_OPIL_INITIALIZE_CONTROL", "OCP_IF_CMD_OPIL_GET_CONTROL", "OCP_IF_CMD_OPIL_GET_CONTROLLER_DATA", "OCP_IF_CMD_END"] ("CMD")
                    n146 = shared-variable ".\\Share_Variables.lvlib\\number_signals"(w409) -> ()  [unwired: 1 in, 1 out]
                    n147 = call "Fc_TCP_Client_33.vi"("CMD"=w412, "Input Cluster"=w410, "error in (no error)"=w413, "Comunication Cluster"=w411) -> ("Output cluster"=w416:T11, "error out"=w414:errorcluster)  [unwired: 4 in, 1 out]
                    n148 = call <vilib>:"Simple Error Handler.vi"("error in (no error)"=w414) -> ()  [unwired: 4 in, 5 out]
                    n149 = Unbundle By Name(w416) -> ("NAMES TRACED SIGNALS"=w415:string[])
                    n150 = Bundle By Name(cluster=w418, "NB_SIGNALS"=w409, "SIGNALS_NAMES"=w415) -> (w417:T3)
                    n151 = shared-variable ".\\Share_Variables.lvlib\\Signals_name"(w415) -> ()  [unwired: 1 in, 1 out]
                  }
                }
              }
            }
            n152 = shared-variable ".\\Share_Variables.lvlib\\Mode_signal_conf"("Mode") -> ()  [unwired: 1 in, 1 out]
            n153 = case shown="\"Item 0\", Default" "Mode" {
              tunnel: [200 ("Refresh time (sec)") w420] -> w363
              frame "Item 1" {
              }
              frame "Item 0", Default {
                n154 = Multiply(x=1, y="Refresh \ntime (ms)") -> (x*y=w420:i32)
              }
            }
            n155 = Bundle By Name(cluster=w358, "Refresh time ms"=w363, "Mode"="Mode", "Start"=TRUE, "DATA"=w354) -> (w365:T3)
          }
        }
      }
      event "Trace names", "# Control": Value Change {
        n156 = event-data() -> ()  [unwired: 1 in, 6 out]
        n157 = Unbundle By Name(w423) -> ("Port"=w431:i32, "hostname"=w430:string, "timeout ms"=w429:i32)
        n158 = Bundle By Name(cluster=w427, "timeout ms"=w429, "remote port"=w431, "Address"=w430) -> (w426:T7)
        n159 = flat-sequence {
          tunnel: w424 -> [w445]
          tunnel: [w445] -> w432
          tunnel: [w447] -> w428
          tunnel: w426 -> [w446]
          tunnel: [w446] -> w425
          tunnel: [w458] -> w433
          tunnel: w432 -> [w462]
          tunnel: w428 -> [w457]
          tunnel: w425 -> [w456]
          frame #0 {
            w448 = 2 items=["OCP_IF_CMD_TRACE_READ", "OCP_IF_CMD_TRACE_RESET", "OCP_IF_CMD_TRACE_GET_SIZE", "OCP_IF_CMD_TRACE_SET_SIZE", "OCP_IF_CMD_TRACE_GET_NUMBER_SIGNALS", "OCP_IF_CMD_TRACE_GET_SIGNALS_NAMES", "OCP_IF_CMD_TRACE_GET_NUMBER_TRACES", "OCP_IF_CMD_TRACE_GET_TRACES_NAMES", "OCP_IF_CMD_TRACE_GET_ADDRESS", "OCP_IF_CMD_CS_STATUS", "OCP_IF_CMD_CS_ENABLE", "OCP_IF_CMD_CS_DISABLE", "OCP_IF_CMD_CS_CONTROLLER_IF", "OCP_IF_CMD_CS_HARDWARE_IF", "OCP_IF_CMD_CS_GET_NUMBER_CONTROLLERS", "OCP_IF_CMD_CS_GET_CONTROLLERS_NAMES", "OCP_IF_CMD_PLATFORM_ID", "OCP_IF_CMD_PLATFORM_IF", "OCP_IF_CMD_OPIL_UPDATE_MEASUREMENTS", "OCP_IF_CMD_OPIL_UPDATE_SIM_DATA", "OCP_IF_CMD_OPIL_RUN_CONTROL", "OCP_IF_CMD_OPIL_INITIALIZE_CONTROL", "OCP_IF_CMD_OPIL_GET_CONTROL", "OCP_IF_CMD_OPIL_GET_CONTROLLER_DATA", "OCP_IF_CMD_END"] ("CMD")
            n160 = property on="Trace names" class="CmbBox"() -> ("Value"=w440:string, "Strings[]"=w441:string[])  [unwired: 2 in, 2 out]
            n161 = Search 1D Array(1D array=w441, element=w440) -> (index of element=w436:i32)  [unwired: 1 in]
            n162 = Less Than 0?(x=w436) -> (x < 0?=w437:bool)
            n163 = Select(t=0, s=w437, f=w436) -> (s? t:f=w435:i32)
            n164 = To Long Integer(number=w435) -> (32bit integer=w439:i32)
            n165 = Bundle By Name(cluster=w445, "TRACE ID"=w439) -> (w444:T6)
            n166 = call "Fc_TCP_Client_33.vi"("CMD"=w448, "Input Cluster"=w444, "Comunication Cluster"=w446) -> ("Output cluster"=w442:T11, "error out"=w447:errorcluster)  [unwired: 5 in, 1 out]
            n167 = Unbundle By Name(w442) -> ("TRACE_SIZE"=w443:i32)
            n168 = property on="Size bytes X #Traces" class="DigNum (strict)"("Value"=w443) -> ()  [unwired: 2 in, 2 out]
          }
          frame #1 {
            w461 = 9 items=["OCP_IF_CMD_TRACE_READ", "OCP_IF_CMD_TRACE_RESET", "OCP_IF_CMD_TRACE_GET_SIZE", "OCP_IF_CMD_TRACE_SET_SIZE", "OCP_IF_CMD_TRACE_GET_NUMBER_SIGNALS", "OCP_IF_CMD_TRACE_GET_SIGNALS_NAMES", "OCP_IF_CMD_TRACE_GET_NUMBER_TRACES", "OCP_IF_CMD_TRACE_GET_TRACES_NAMES", "OCP_IF_CMD_TRACE_GET_ADDRESS", "OCP_IF_CMD_CS_STATUS", "OCP_IF_CMD_CS_ENABLE", "OCP_IF_CMD_CS_DISABLE", "OCP_IF_CMD_CS_CONTROLLER_IF", "OCP_IF_CMD_CS_HARDWARE_IF", "OCP_IF_CMD_CS_GET_NUMBER_CONTROLLERS", "OCP_IF_CMD_CS_GET_CONTROLLERS_NAMES", "OCP_IF_CMD_PLATFORM_ID", "OCP_IF_CMD_PLATFORM_IF", "OCP_IF_CMD_OPIL_UPDATE_MEASUREMENTS", "OCP_IF_CMD_OPIL_UPDATE_SIM_DATA", "OCP_IF_CMD_OPIL_RUN_CONTROL", "OCP_IF_CMD_OPIL_INITIALIZE_CONTROL", "OCP_IF_CMD_OPIL_GET_CONTROL", "OCP_IF_CMD_OPIL_GET_CONTROLLER_DATA", "OCP_IF_CMD_END"] ("CMD")
            # "pending to define"
            n169 = property on="# Control" class="CmbBox"() -> ("Value"=w454:string, "Strings[]"=w455:string[])  [unwired: 2 in, 2 out]
            n170 = Search 1D Array(1D array=w455, element=w454) -> (index of element=w451:i32)  [unwired: 1 in]
            n171 = Less Than 0?(x=w451) -> (x < 0?=w453:bool)
            n172 = Select(t=0, s=w453, f=w451) -> (s? t:f=w450:i32)
            n173 = To Long Integer(number=w450) -> (32bit integer=w449:i32)
            n174 = Bundle By Name(cluster=w462, "CS_ID"=w449) -> (w459:T6)
            n175 = call "Fc_TCP_Client_33.vi"("CMD"=w461, "Input Cluster"=w459, "error in (no error)"=w457, "Comunication Cluster"=w456) -> ("Output cluster"=w463:T11, "error out"=w458:errorcluster)  [unwired: 4 in, 1 out]
            n176 = Unbundle By Name(w463) -> ("CS STATUS"=→"Current CS status":i32)
          }
        }
        n177 = call <vilib>:"Simple Error Handler.vi"("error in (no error)"=w433) -> ()  [unwired: 4 in, 5 out]
      }
      event "CS enable": Value Change {
        n178 = event-data() -> ()  [unwired: 1 in, 6 out]
        n179 = Unbundle By Name(w465) -> ("Port"=w470:i32, "hostname"=w472:string, "timeout ms"=w471:i32)
        n180 = Bundle By Name(cluster=w475, "timeout ms"=w471, "remote port"=w470, "Address"=w472) -> (w473:T7)
        n181 = flat-sequence {
          tunnel: w474 -> [w484]
          tunnel: w473 -> [w482]
          tunnel: ["CS enable"] -> w469
          tunnel: [w482] -> w468
          tunnel: [w481] -> w467
          tunnel: [w476] -> w464
          tunnel: w469 -> [w498]
          tunnel: w468 -> [w496]
          tunnel: w467 -> [w497]
          tunnel: w465 -> [w494]
          tunnel: [w493] -> w466
          tunnel: w464 -> [w492]
          frame #0 {
            n182 = property on="# Control" class="CmbBox"() -> ("Value"=w485:string, "Strings[]"=w486:string[])  [unwired: 2 in, 2 out]
            n183 = Search 1D Array(1D array=w486, element=w485) -> (index of element=w479:i32)  [unwired: 1 in]
            n184 = Less Than 0?(x=w479) -> (x < 0?=w480:bool)
            n185 = Select(t=0, s=w480, f=w479) -> (s? t:f=w477:i32)
            n186 = To Long Integer(number=w477) -> (32bit integer=w476:i32)
            n187 = Bundle By Name(cluster=w484, "CS_ID"=w476) -> (w481:T6)
          }
          frame #1 {
            n188 = case shown="False" w498 {
              selector: w498 -> [w500 w510]
              tunnel: w496 -> [w504 w515]
              tunnel: w497 -> [w501 w512]
              tunnel: [w502 w513] -> w495
              tunnel: [w500 w509] -> w490
              tunnel: w492 -> [_ w508]
              tunnel: [0 w508] -> w491
              frame False {
                w503 = 11 items=["OCP_IF_CMD_TRACE_READ", "OCP_IF_CMD_TRACE_RESET", "OCP_IF_CMD_TRACE_GET_SIZE", "OCP_IF_CMD_TRACE_SET_SIZE", "OCP_IF_CMD_TRACE_GET_NUMBER_SIGNALS", "OCP_IF_CMD_TRACE_GET_SIGNALS_NAMES", "OCP_IF_CMD_TRACE_GET_NUMBER_TRACES", "OCP_IF_CMD_TRACE_GET_TRACES_NAMES", "OCP_IF_CMD_TRACE_GET_ADDRESS", "OCP_IF_CMD_CS_STATUS", "OCP_IF_CMD_CS_ENABLE", "OCP_IF_CMD_CS_DISABLE", "OCP_IF_CMD_CS_CONTROLLER_IF", "OCP_IF_CMD_CS_HARDWARE_IF", "OCP_IF_CMD_CS_GET_NUMBER_CONTROLLERS", "OCP_IF_CMD_CS_GET_CONTROLLERS_NAMES", "OCP_IF_CMD_PLATFORM_ID", "OCP_IF_CMD_PLATFORM_IF", "OCP_IF_CMD_OPIL_UPDATE_MEASUREMENTS", "OCP_IF_CMD_OPIL_UPDATE_SIM_DATA", "OCP_IF_CMD_OPIL_RUN_CONTROL", "OCP_IF_CMD_OPIL_INITIALIZE_CONTROL", "OCP_IF_CMD_OPIL_GET_CONTROL", "OCP_IF_CMD_OPIL_GET_CONTROLLER_DATA", "OCP_IF_CMD_END"] ("CMD")
                n189 = call "Fc_TCP_Client_33.vi"("CMD"=w503, "Input Cluster"=w501, "Comunication Cluster"=w504) -> ("error out"=w502:errorcluster)  [unwired: 5 in, 2 out]
              }
              frame True {
                w514 = 10 items=["OCP_IF_CMD_TRACE_READ", "OCP_IF_CMD_TRACE_RESET", "OCP_IF_CMD_TRACE_GET_SIZE", "OCP_IF_CMD_TRACE_SET_SIZE", "OCP_IF_CMD_TRACE_GET_NUMBER_SIGNALS", "OCP_IF_CMD_TRACE_GET_SIGNALS_NAMES", "OCP_IF_CMD_TRACE_GET_NUMBER_TRACES", "OCP_IF_CMD_TRACE_GET_TRACES_NAMES", "OCP_IF_CMD_TRACE_GET_ADDRESS", "OCP_IF_CMD_CS_STATUS", "OCP_IF_CMD_CS_ENABLE", "OCP_IF_CMD_CS_DISABLE", "OCP_IF_CMD_CS_CONTROLLER_IF", "OCP_IF_CMD_CS_HARDWARE_IF", "OCP_IF_CMD_CS_GET_NUMBER_CONTROLLERS", "OCP_IF_CMD_CS_GET_CONTROLLERS_NAMES", "OCP_IF_CMD_PLATFORM_ID", "OCP_IF_CMD_PLATFORM_IF", "OCP_IF_CMD_OPIL_UPDATE_MEASUREMENTS", "OCP_IF_CMD_OPIL_UPDATE_SIM_DATA", "OCP_IF_CMD_OPIL_RUN_CONTROL", "OCP_IF_CMD_OPIL_INITIALIZE_CONTROL", "OCP_IF_CMD_OPIL_GET_CONTROL", "OCP_IF_CMD_OPIL_GET_CONTROLLER_DATA", "OCP_IF_CMD_END"] ("CMD")
                n190 = call "Fc_TCP_Client_33.vi"("CMD"=w514, "Input Cluster"=w512, "Comunication Cluster"=w515) -> ("Output cluster"=w511:T11, "error out"=w513:errorcluster)  [unwired: 5 in, 1 out]
                n191 = Unbundle By Name(w511) -> ("SIZE"=w507:i32)
                n192 = Not A Number/Path/Refnum?(number/path/refnum=w507) -> (NaN/Path/Refnum?=w506:bool)
                n193 = Not(x=w506) -> (.not. x?=w505:bool)
                n194 = And(x=w505, y=w510) -> (x .and. y?=w509:bool)
              }
            }
            n195 = Bundle By Name(cluster=w494, "CS enable?"=w490, "CS ID"=w491) -> (w493:T3)
            n196 = Select(t=cluster{u32, u32}[] [{3381759, 3381759}] ("Colors [4]"), s=w490, f=cluster{u32, u32}[] [{11776947, 11776947}] ("Colors [4]")) -> (s? t:f=w489:cluster{u32, u32}[])
            n197 = property on="CS enable" class="Bool (strict)"("Colors [4]"=w489) -> ()  [unwired: 2 in, 2 out]
            n198 = call <vilib>:"Simple Error Handler.vi"("error in (no error)"=w495) -> ()  [unwired: 4 in, 5 out]
          }
        }
      }
      event "Save CTRL parameters": Value Change {
        n199 = event-data() -> ()  [unwired: 1 in, 6 out]
        n200 = Unbundle By Name(w531) -> ("Port"=w527:i32, "hostname"=w526:string, "timeout ms"=w525:i32, "CS enable?"=w517:bool, "CS ID"=w518:i32)
        n201 = Bundle By Name(cluster=w528, "timeout ms"=w525, "remote port"=w527, "Address"=w526) -> (w524:T7)
        n202 = Bundle By Name(cluster=w523, "CS_ID"=w518) -> (w519:T5)
        n203 = And(x="Save CTRL parameters", y=w517) -> (x .and. y?=w529:bool)
        n204 = case shown="True" w529 {
          selector: w529 -> [w536 w554]
          tunnel: w524 -> [w553 _]
          tunnel: w532 -> [w551 w555]
          tunnel: w519 -> [w552 _]
          tunnel: [w550 w555] -> w522
          tunnel: "CS_IF_Params" -> [w549 _]
          tunnel: T10."little-endian" ("byte order (0:big-endian, network order)") -> [w548 _]
          tunnel: [w535 w554] -> w516
          frame True {
            w547 = 12 items=["OCP_IF_CMD_TRACE_READ", "OCP_IF_CMD_TRACE_RESET", "OCP_IF_CMD_TRACE_GET_SIZE", "OCP_IF_CMD_TRACE_SET_SIZE", "OCP_IF_CMD_TRACE_GET_NUMBER_SIGNALS", "OCP_IF_CMD_TRACE_GET_SIGNALS_NAMES", "OCP_IF_CMD_TRACE_GET_NUMBER_TRACES", "OCP_IF_CMD_TRACE_GET_TRACES_NAMES", "OCP_IF_CMD_TRACE_GET_ADDRESS", "OCP_IF_CMD_CS_STATUS", "OCP_IF_CMD_CS_ENABLE", "OCP_IF_CMD_CS_DISABLE", "OCP_IF_CMD_CS_CONTROLLER_IF", "OCP_IF_CMD_CS_HARDWARE_IF", "OCP_IF_CMD_CS_GET_NUMBER_CONTROLLERS", "OCP_IF_CMD_CS_GET_CONTROLLERS_NAMES", "OCP_IF_CMD_PLATFORM_ID", "OCP_IF_CMD_PLATFORM_IF", "OCP_IF_CMD_OPIL_UPDATE_MEASUREMENTS", "OCP_IF_CMD_OPIL_UPDATE_SIM_DATA", "OCP_IF_CMD_OPIL_RUN_CONTROL", "OCP_IF_CMD_OPIL_INITIALIZE_CONTROL", "OCP_IF_CMD_OPIL_GET_CONTROL", "OCP_IF_CMD_OPIL_GET_CONTROLLER_DATA", "OCP_IF_CMD_END"] ("CMD")
            n205 = Unbundle By Name(w549) -> ("SET_PARAMETERS"=w544:i32, "CTLR"=w543:i32, "CS_Duty"=w542:sgl)
            n206 = Wait (ms)(milliseconds to wait=u32 200) -> ()  [unwired: 1 out]
            n207 = Flatten To String(anything=w544, prepend array or string size? (T)=w536, byte order (0:big-endian, network order)=w548, error in (no error)=w551) -> (data string=w541:string, error out=w546:errorcluster)  [unwired: 1 out]
            n208 = Flatten To String(anything=w543, prepend array or string size? (T)=w536, byte order (0:big-endian, network order)=w548, error in (no error)=w546) -> (data string=w540:string, error out=w545:errorcluster)  [unwired: 1 out]
            n209 = Flatten To String(anything=w542, prepend array or string size? (T)=w536, byte order (0:big-endian, network order)=w548, error in (no error)=w545) -> (data string=w539:string, error out=w534:errorcluster)  [unwired: 1 out]
            n210 = Concatenate Strings(w541, w540, w539) -> (w537:string)
            n211 = Not(x=w536) -> (.not. x?=w535:bool)
            n212 = Bundle By Name(cluster=w552, "DATA PARAM"=w537) -> (w538:T5)
            n213 = call "Fc_TCP_Client_34.vi"("CMD"=w547, "Input Cluster"=w538, "error in (no error)"=w534, "Comunication Cluster"=w553) -> ("error out"=w550:errorcluster)  [unwired: 4 in, 2 out]
          }
          frame False {
          }
        }
        n214 = call <vilib>:"Simple Error Handler.vi"("error in (no error)"=w522) -> ()  [unwired: 4 in, 5 out]
        n215 = local write "Save CTRL parameters"(w516) -> ()
      }
      event "CTRL enable": Value Change {
        w561 = TRUE
        w568 = 12 items=["OCP_IF_CMD_TRACE_READ", "OCP_IF_CMD_TRACE_RESET", "OCP_IF_CMD_TRACE_GET_SIZE", "OCP_IF_CMD_TRACE_SET_SIZE", "OCP_IF_CMD_TRACE_GET_NUMBER_SIGNALS", "OCP_IF_CMD_TRACE_GET_SIGNALS_NAMES", "OCP_IF_CMD_TRACE_GET_NUMBER_TRACES", "OCP_IF_CMD_TRACE_GET_TRACES_NAMES", "OCP_IF_CMD_TRACE_GET_ADDRESS", "OCP_IF_CMD_CS_STATUS", "OCP_IF_CMD_CS_ENABLE", "OCP_IF_CMD_CS_DISABLE", "OCP_IF_CMD_CS_CONTROLLER_IF", "OCP_IF_CMD_CS_HARDWARE_IF", "OCP_IF_CMD_CS_GET_NUMBER_CONTROLLERS", "OCP_IF_CMD_CS_GET_CONTROLLERS_NAMES", "OCP_IF_CMD_PLATFORM_ID", "OCP_IF_CMD_PLATFORM_IF", "OCP_IF_CMD_OPIL_UPDATE_MEASUREMENTS", "OCP_IF_CMD_OPIL_UPDATE_SIM_DATA", "OCP_IF_CMD_OPIL_RUN_CONTROL", "OCP_IF_CMD_OPIL_INITIALIZE_CONTROL", "OCP_IF_CMD_OPIL_GET_CONTROL", "OCP_IF_CMD_OPIL_GET_CONTROLLER_DATA", "OCP_IF_CMD_END"] ("CMD")
        w574 = T10."little-endian" ("byte order (0:big-endian, network order)")
        n216 = event-data() -> ()  [unwired: 1 in, 6 out]
        n217 = Unbundle By Name(w582) -> ("Port"=w580:i32, "hostname"=w579:string, "timeout ms"=w578:i32, "CS enable?"=w572:bool, "CS ID"=w573:i32)
        n218 = Bundle By Name(cluster=w581, "timeout ms"=w578, "remote port"=w580, "Address"=w579) -> (w577:T7)
        n219 = Bundle By Name(cluster=w576, "CS_ID"=w573) -> (w570:T5)
        n220 = local read "CS_IF_Params"() -> (w569:T2)
        n221 = And(x="CTRL enable", y=w572) -> (x .and. y?=w559:bool)
        n222 = Unbundle By Name(w569) -> ("CTRL_IF_SET"=w560:i32)
        n223 = Flatten To String(anything=w560, prepend array or string size? (T)=w561, byte order (0:big-endian, network order)=w574, error in (no error)=w583) -> (data string=w566:string, error out=w567:errorcluster)  [unwired: 1 out]
        n224 = Select(t=2 ("CTRL_IF_SET"), s=w559, f=0 ("CTRL_IF_SET")) -> (s? t:f=w557:i32)
        n225 = Flatten To String(anything=w557, prepend array or string size? (T)=w561, byte order (0:big-endian, network order)=w574, error in (no error)=w567) -> (data string=w565:string, error out=w564:errorcluster)  [unwired: 1 out]
        n226 = Concatenate Strings(w566, w565) -> (w563:string)
        n227 = Bundle By Name(cluster=w570, "DATA PARAM"=w563) -> (w562:T5)
        n228 = call "Fc_TCP_Client_34.vi"("CMD"=w568, "Input Cluster"=w562, "error in (no error)"=w564, "Comunication Cluster"=w577) -> ("error out"=w575:errorcluster)  [unwired: 4 in, 2 out]
        n229 = call <vilib>:"Simple Error Handler.vi"("error in (no error)"=w575) -> ()  [unwired: 4 in, 5 out]
      }
    }
    n230 = property on="Multicolumn Listbox" class="MCListbox (strict)"() -> ("ItemNames"=w56:string[][])  [unwired: 2 in, 2 out]
    n231 = Index Array(array=w53, index=0) -> (element=w52:refnum<queue>)
    n232 = case shown="True" "Send message" {
      tunnel: w56 -> [_ w74]
      tunnel: w55 -> [_ w76]
      tunnel: w52 -> [_ w75]
      frame False {
      }
      frame True {
        n233 = Array Size(array=w74) -> (size(s)=w72:i32[])
        n234 = case shown="Default" "Process 2" {
          selector: "Process 2" -> [w94 _]
          tunnel: w74 -> [w96 _]
          tunnel: w76 -> [w84 _]
          tunnel: w75 -> [w85 _]
          frame Default {
            w80 = FALSE ("create if not found? (T)")
            n235 = Get Queue Status(queue=w85, error in (no error)=w84) -> (error out=w82:errorcluster)  [unwired: 1 in, 7 out]
            n236 = Index Array(array=w96, index (row)=w94, index (col)=0 ("disabled index (col)")) -> (element=w78:string)
            n237 = local write "Send message"(w80) -> ()
            n238 = Obtain Queue(name (unnamed)=w78, element data type="", create if not found? (T)=w80, error in (no error)=w82) -> (queue out=w83:refnum<queue>, error out=w81:errorcluster)  [unwired: 1 in, 1 out]
            n239 = Concatenate Strings("message::", "msj") -> (w89:string)
            n240 = Get Queue Status(queue=w83, error in (no error)=w81) -> (queue out=w93:refnum<queue>, error out=w92:errorcluster)  [unwired: 1 in, 6 out]
            n241 = Enqueue Element(queue=w93, element=w89, error in (no error)=w92) -> (queue out=w88:refnum<queue>, error out=w87:errorcluster)  [unwired: 1 in, 1 out]
            n242 = Release Queue(queue=w88, error in (no error)=w87) -> (error out=w86:errorcluster)  [unwired: 1 in, 2 out]
            n243 = call <vilib>:"Simple Error Handler.vi"("error in (no error)"=w86) -> ()  [unwired: 4 in, 5 out]
          }
          frame ..-1 {
          }
        }
        n244 = Index Array(array=w72, index=0) -> (element=w71:i32)
        n245 = property on="Process 2" class="DigNum (strict)"("Maximum"=w71) -> ()  [unwired: 2 in, 2 out]
      }
    }
    n246 = Dequeue Element(queue=w68, timeout in ms (-1)=100, error in (no error)=w64) -> (queue out=w65:refnum<queue>, element=w67:string, timed out?=w66:bool, error out=w58:errorcluster)
    n247 = case shown="False" w66 {
      tunnel: w67 -> [w99 _]
      frame False {
        n248 = Match Pattern(string=w99, regular expression="::") -> (before substring=w98:string, after substring=w97:string)  [unwired: 1 in, 2 out]
        n249 = case shown="\"process started\"" w98 {
          tunnel: w97 -> [_ w109 w114]
          frame "False", Default {
            # "unhandled received commands."
            n250 = call <vilib>:"Error Cluster From Error Code.vi"("error message (\"\")"="Invalid command received from process VI" ("error message (\"\")"), "error code (0)"=1) -> ("error out"=w101:errorcluster)  [unwired: 7 in]
            n251 = call <vilib>:"Simple Error Handler.vi"("error in (no error)"=w101) -> ()  [unwired: 4 in, 5 out]
          }
          frame "process stopped" {
            n252 = property on="Multicolumn Listbox" class="MCListbox (strict)"() -> ("ItemNames"=w105:string[][])  [unwired: 2 in, 2 out]
            n253 = Index Array(array=w105, index (col)=0 ("disabled index (col)")) -> (element=w106:string[])  [unwired: 1 in]
            n254 = Search 1D Array(1D array=w106, element=w109) -> (index of element=w107:i32)  [unwired: 1 in]
            n255 = Delete From Array(array=w105, index (row)=w107) -> (array with subset deleted=w104:string[][])  [unwired: 2 in, 1 out]
            n256 = property on="Multicolumn Listbox" class="MCListbox (strict)"("ItemNames"=w104) -> ()  [unwired: 2 in, 2 out]
          }
          frame "process started" {
            n257 = Build Array(w114, "" ("element")) -> (w112:string[])
            n258 = property on="Multicolumn Listbox" class="MCListbox (strict)"() -> ("ItemNames"=w111:string[][])  [unwired: 2 in, 2 out]
            n259 = Build Array (concatenate)(w111, w112) -> (w110:string[][])
            n260 = property on="Multicolumn Listbox" class="MCListbox (strict)"("ItemNames"=w110) -> ()  [unwired: 2 in, 2 out]
          }
        }
      }
      frame True {
      }
    }
  }
  n261 = invoke on="Size bytes X #Traces" class="DigNum (strict)" method="Reinit To Default"(error in=w15) -> (error out=w14:errorcluster)  [unwired: 2 in, 2 out]
  n262 = shared-variable ".\\Share_Variables.lvlib\\Close_all_wplots"(FALSE ("Close_all_wplots"), error in=w14) -> (error out=w20:errorcluster)
  n263 = invoke on="Multicolumn Listbox" class="MCListbox (strict)" method="Reinit To Default"(error in=w20) -> (error out=w29:errorcluster)  [unwired: 2 in, 2 out]
  n264 = property on="Multicolumn Listbox" class="MCListbox (strict)"(error in=w29, "ItemNames"=string[][] [] ("Item Names")) -> (error out=w13:errorcluster)  [unwired: 1 in, 1 out]
  n265 = property on="New plot" class="Bool (strict)"(error in=w13, "Value"=FALSE ("New plot"), "Visible"=TRUE, "DisabledEnum"=T4."Enabled" ("Disabled")) -> (error out=w12:errorcluster)  [unwired: 1 in, 1 out]
  n266 = property on="Close All plots" class="Bool (strict)"(error in=w12, "Value"=FALSE ("Cancel Button")) -> (error out=w7:errorcluster)  [unwired: 1 in, 1 out]
  n267 = invoke on="Waveform Chart 2" class="WFChart (strict)" method="Reinit To Default"(error in=w7) -> (error out=w6:errorcluster)  [unwired: 2 in, 2 out]
  n268 = shared-variable ".\\Share_Variables.lvlib\\Signals_value_Array"(dbl[] [] ("Signals_value_Array"), error in=w6) -> (error out=w5:errorcluster)
  n269 = property on="CS enable" class="Bool (strict)"(error in=w5, "Colors [4]"=cluster{u32, u32}[] [{11776947, 11776947}]) -> (error out=w3:errorcluster)  [unwired: 1 in, 1 out]
  n270 = property on="Refresh \ntime (ms)" class="DigNum (strict)"(error in=w3, "Value"=500 ("Refresh \ntime (ms)")) -> (error out=w2:errorcluster)  [unwired: 1 in, 1 out]
  n271 = call <vilib>:"Simple Error Handler.vi"("error in (no error)"=w2) -> ()  [unwired: 4 in, 5 out]
  n272 = Flush Queue(queue=w31) -> ()  [unwired: 1 in, 3 out]
  n273 = for {
    tunnel: w45 -> [w585] mode=indexing
    n274 = Release Queue(queue=w585, force destroy? (F)=FALSE) -> ()  [unwired: 1 in, 3 out]
  }
  n275 = Release Queue(queue=w31, error in (no error)=w40) -> (error out=w38:errorcluster)  [unwired: 1 in, 2 out]
  n276 = property on="Multicolumn Listbox" class="MCListbox (strict)"(error in=w38) -> (error out=w34:errorcluster, "ItemNames"=w37:string[][])  [unwired: 1 in, 1 out]
  n277 = Index Array(array=w37, index (col)=0 ("disabled index (col)")) -> (element=w35:string[])  [unwired: 1 in]
  n278 = for {
    tunnel: w35 -> [w595] mode=indexing
    shift-right: [w592] -> w33
    shift-left: w34 -> [w594]
    n279 = Obtain Queue(name (unnamed)=w595, element data type="", error in (no error)=w594) -> (queue out=w587:refnum<queue>, error out=w589:errorcluster)  [unwired: 2 in, 1 out]
    n280 = Enqueue Element(queue=w587, element="exit::", error in (no error)=w589) -> (queue out=w586:refnum<queue>, error out=w588:errorcluster)  [unwired: 1 in, 1 out]
    n281 = Release Queue(queue=w586, force destroy? (F)=FALSE, error in (no error)=w588) -> (error out=w592:errorcluster)  [unwired: 2 out]
  }
  n282 = call <vilib>:"Simple Error Handler.vi"("error in (no error)"=w33) -> ("error out"=w32:errorcluster)  [unwired: 4 in, 4 out]
  n283 = flat-sequence {
    tunnel: w32 -> [_]
    frame #0 {
      n284 = property class="App"() -> ("App.Kind"=w598:T12)  [unwired: 2 in, 2 out]
      n285 = Equal?(x=w598, y=T12."Run Time System" ("Application:Kind")) -> (x = y?=→"Close":bool)
    }
  }
